vi "OAXML_Save Header.vi"(8 "file name":string, 9 "Param in":T3, 10 "tacho channel index":i32, 11 "DAQ Config":T1 {"pregain" format="%.2f"; "IEPE" items=["On", "Off", "None"]; "coupling" items=["DC", "AC"]; "engineering units" items=["custom..."=0, "V"=1, "A"=21, "C"=30, "pC"=31, "s"=32, "-"=29, "Pa"=2, "N"=20, "g"=3, "m/s^2"=4, "m/s"=5, "m"=6, "mm/s"=12, "mm"=13, "micron/s"=14, "micron"=15, "in/s^2"=7, "in/s"=8, "in"=9, "mil/s"=10, "mil"=11, "rad/s^2"=16, "rad/s"=17, "rad"=18, "deg/s^2"=26, "deg/s"=27, "deg"=28, "RPM"=22, "cycle/s^2"=23, "Hz"=24, "cycle"=25, "strain"=19]; "sensor sensitivity (mV/EU)" format="%.2f"; "dB reference" format="%.1e"}) -> (3 "file refnum":refnum<file>)   [LabVIEW 2017]
uses:
  <vilib>/addons/Sound and Vibration/Order Analysis/Example Support/sub VIs/OAXML_DSA DAQ Config.ctl
  <vilib>/addons/_NISVFA/_Shared subVIs/Controls/svc_Engineering Units Text Ring.ctl
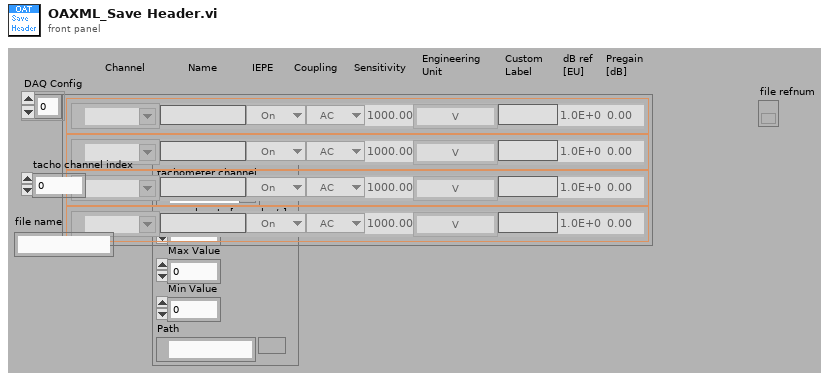
[diagram p1: front panel]
types:
  T1 = typedef "OAXML_DSA DAQ Config.ctl" = cluster{"name":string, "channel":tag, "coupling":u16, "dB reference":sgl, "sensor sensitivity (mV/EU)":dbl, "engineering units":T2, "IEPE":u16, "custom label":string, "pregain":sgl}[]
  T2 = typedef "svc_Engineering Units Text Ring.ctl" = u16
  T3 = cluster{"tachometer channel":tag, "sample rate [samples/s]":dbl, "Max Value":dbl, "Min Value":dbl, "Path":path}
  T4 = enum16{"open", "open or create", "create or replace", "create", "open (read only)"}
  T5 = cluster{"name":string, "channel":tag, "coupling":u16, "dB reference":sgl, "sensor sensitivity (mV/EU)":dbl, "engineering units":T2, "IEPE":u16, "custom label":string, "pregain":sgl}
  T6 = cluster{"name":string, "sample rate [samples/s]":dbl, "sample rate [samples/s]":dbl, "sensor sensitivity (mV/EU)":dbl, "engineering units":T2}
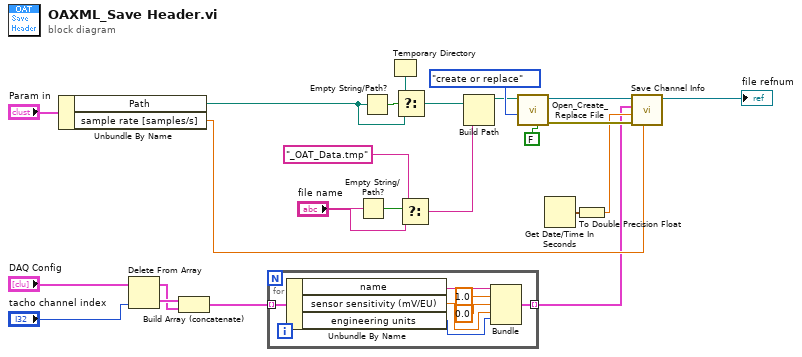
[diagram p0: block diagram]
diagram:
  n1 = Unbundle By Name("Param in") -> ("Path"=w7:path, "sample rate [samples/s]"=w8:dbl)
  n2 = Delete From Array(array="DAQ Config", index="tacho channel index") -> (deleted portion=w4:T5, array with subset deleted=w3:T1)  [unwired: 1 in]
  n3 = Build Array (concatenate)(w4, w3) -> (w2:T1)
  n4 = for {
    tunnel: w2 -> [w31] mode=indexing
    tunnel: [w25] -> w1 mode=indexing
    n5 = Unbundle By Name(w31) -> ("name"=w30:string, "sensor sensitivity (mV/EU)"=w27:dbl, "engineering units"=w26:T2)
    n6 = Bundle("name"=w30, "sample rate [samples/s]"=1.0, "sample rate [samples/s]"=0.0, "sensor sensitivity (mV/EU)"=w27, "engineering units"=w26) -> (w25:T6)  [unwired: 1 in]
  }
  n7 = Empty String/Path?(string/path="file name") -> (empty?=w16:bool)
  n8 = Empty String/Path?(string/path=w7) -> (empty?=w17:bool)
  n9 = Temporary Directory() -> (w19:path)
  n10 = Select(t=w19, s=w17, f=w7) -> (s? t:f=w18:path)
  n11 = Select(t="_OAT_Data.tmp" ("time format string (%c)"), s=w16, f="file name") -> (s? t:f=w14:string)
  n12 = Build Path(base path=w18, name or relative path=w14) -> (appended path=w22:path)
  n13 = call <vilib>:"Open_Create_Replace File.vi"("advisory dialog? (display:T)"=FALSE, "function (open:0)"=T4."create or replace", "file path"=w22) -> ("error out"=w20:errorcluster, "refnum"=w21:refnum<file>)  [unwired: 5 in, 2 out]
  n14 = Get Date/Time In Seconds() -> (seconds since 1Jan1904=w10:timestamp)
  n15 = To Double Precision Float(number=w10) -> (double precision float=w11:dbl)
  n16 = call <vilib>:"Save Channel Info.vi"("Sample rate"=w8, "error in"=w20, "time"=w11, "channel info"=w1, "refnum in"=w21) -> ("refnum out"=→"file refnum":refnum<file>)  [unwired: 5 in, 1 out]
